vi "RemoteControl.Configure.vi"(8 "error in (no error)":errorcluster, 10 "Configure":T1, 11 "RemoteControl":refnum<class "RemoteControl.lvclass">) -> (0 "error out":errorcluster, 3 "RemoteControl out":refnum<class "RemoteControl.lvclass">)   [LabVIEW 2019, in "RemoteControl.lvlib" / "RemoteControl.lvclass"]
doc: "---------------------------------------------------------------\nJKI State Machine Objects™\nhttp://jki.net/state-machine-objects/\nCopyright (C) 2005-2015, JKI <info@jki.net>\nALL RIGHTS RESERVEDJKI State Machine Objects (SMO) 1.0.0.4\nJKI - JKI\nCopyright (c) 2015, JKI"
uses:
  RemoteControl.lvclass
  Typedefs/PrivateEvents--RemoteControl.Configure.ctl
  RemoteControl.lvclass/RemoteControl.ctl
panel:
  # "For instructions on how to use the JKI State Machine Objects, examples and video tutorials, visit:\nhttp://jki.net/state-machine-objects/\n\nJKI State Machine Objects™\nhttp://jki.net/state-machine-objects/\nCopyright (C) 2005-2015, JKI <info@jki.net>\nALL RIGHTS RESERVED"
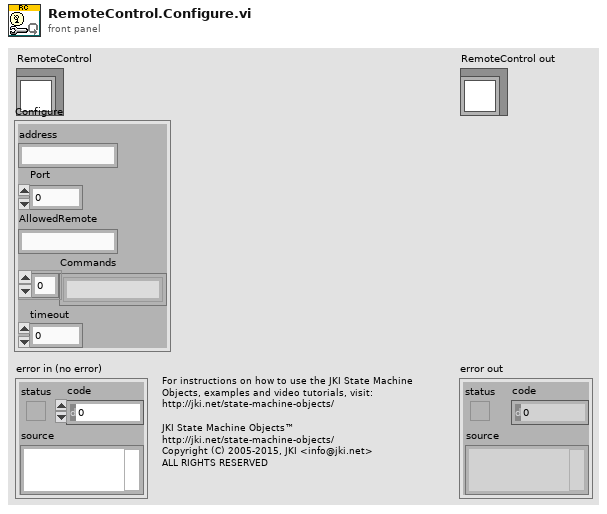
[diagram p1: front panel]
types:
  T1 = typedef "RemoteControl.lvlib/RemoteControl.lvclass/PrivateEvents--RemoteControl.Configure.ctl" = cluster{"address":string, "Port":u16, "AllowedRemote":string, "Commands":string[], "timeout":i32}
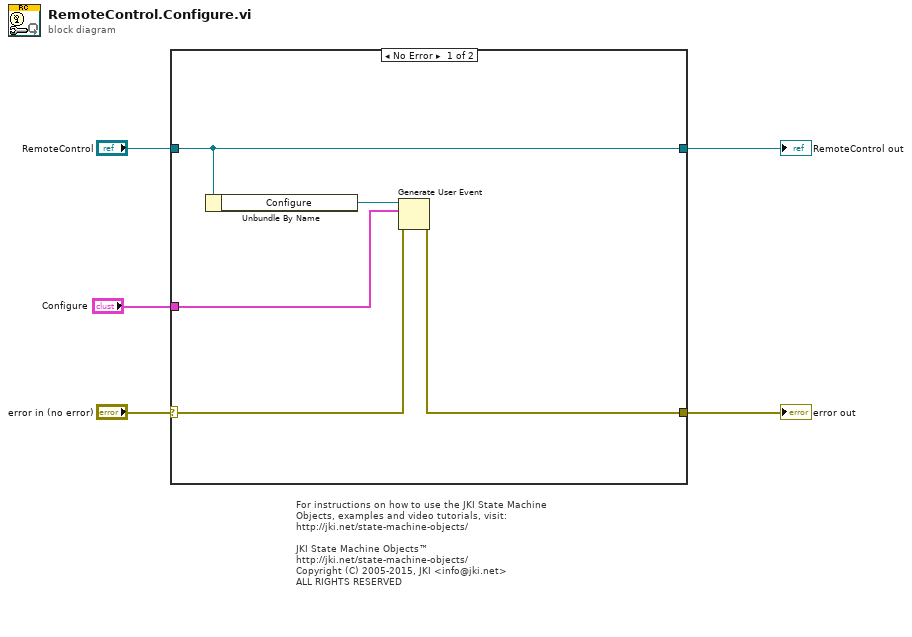
[diagram p0: block diagram]
diagram:
  # "For instructions on how to use the JKI State Machine Objects, examples and video tutorials, visit:\nhttp://jki.net/state-machine-objects/\n\nJKI State Machine Objects™\nhttp://jki.net/state-machine-objects/\nCopyright (C) 2005-2015, JKI <info@jki.net>\nALL RIGHTS RESERVED"
  n1 = case shown="No Error" "error in (no error)" {
    selector: "error in (no error)" -> [w10 w12]
    tunnel: [w8 w12] -> w4
    tunnel: [w6 w11] -> w5
    tunnel: "RemoteControl" -> [w6 w11]
    tunnel: "Configure" -> [w7 _]
    frame No Error {
      n2 = Unbundle By Name(w6) -> ("Configure"=w9:refnum<user-event>)
      n3 = Generate User Event(user event=w9, event data cluster=w7, error in=w10) -> (error out=w8:errorcluster)  [unwired: 1 in, 1 out]
    }
    frame Error {
    }
  }
  "error out" <- w4
  "RemoteControl out" <- w5
